vi "Build XML File Attachment.vi"(8 "error in":errorcluster, 10 "file":path, 11 "Image (false)":bool) -> (0 "error out":errorcluster, 2 "string out (XML Attachment))":string)   [LabVIEW 2013]
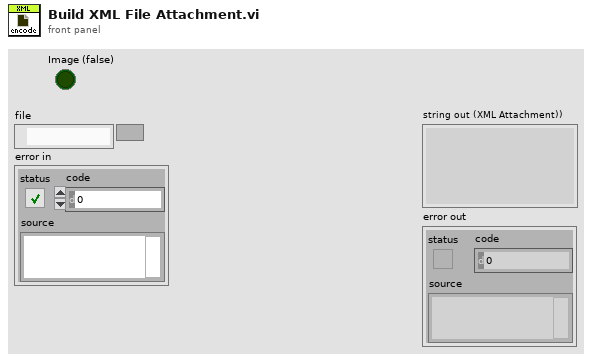
[diagram p1: front panel]
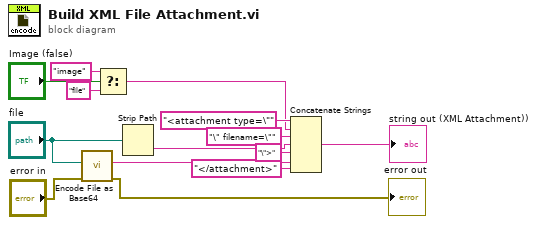
[diagram p0: block diagram]
diagram:
  n1 = call "Encode File as Base64.vi"("error in"="error in", "file"="file") -> ("error out"=→"error out":errorcluster, "string out (base64-encoded)"=w4:string)  [unwired: 8 in]
  n2 = Select(t="image" ("string"), s="Image (false)", f="file" ("string")) -> (s? t:f=w9:string)
  n3 = Strip Path(path="file") -> (name=w6:string)  [unwired: 1 out]
  n4 = Concatenate Strings("<attachment type=\"" ("string"), w9, "\" filename=\"" ("string"), w6, "\">" ("string"), w4, "</attachment>" ("string")) -> (→"string out (XML Attachment))":string)
